vi "Periodic Tasks.vi"(8 "error in":errorcluster) -> ()   [LabVIEW 2016]
doc: "This VI runs in parallel to other tasks. It can contain as many user-defined periodic loops as you need. These can carry out PID or other sorts of timed response."
uses:
  <vilib>/Rock Robotics/WPI/ThirdParty/CanMotor/TalonSRX/WPI_CANTalonSRX_GlobalOps.ctl
  <vilib>/Rock Robotics/WPI/Utilities/WPI_GetSetVariantRefNum.vi
  Robot Global Data.vi
  <vilib>/Rock Robotics/Network Tables/NT Write String Array.vi
  <vilib>/Rock Robotics/Network Tables/NT Write Numeric Array.vi
  2039lib.lvlib
  <vilib>/Rock Robotics/Network Tables/NT Write Number.vi
  <vilib>/Analysis/NI_AALPro.lvlib
  <vilib>/Analysis/2dsp.llb/Integral Method.ctl
  <vilib>/Analysis/8numeric.llb/1D Numeric Integration.vi
panel:
  in  "Auto Names":string[](array[string])
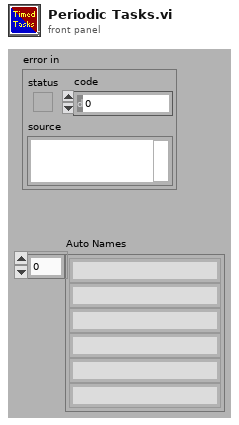
[diagram p1: front panel]
types:
  T1 = typedef "WPI_JoystickDevRef.ctl" = cluster{"Device":T2}
  T2 = typedef "WPI_JoystickDeviceEnum.ctl" = enum16{"USB 0", "USB 1", "USB 2", "USB 3", "USB 4", "USB 5"}
  T3 = typedef "WPI_RobotDriveDevRef.ctl" = cluster{"DevStatus":errorcluster, "Motors[]":T4[], "Square Inputs":bool, "Max Output":dbl}
  T4 = typedef "WPI_MotorControlDeviceRef.ctl" = cluster{"DeviceStatus":errorcluster, "Type":T5, "PWM":cluster{"PWM Channel":T6, "DeadBand":T7}, "CAN":cluster{"Device Number":u8, "SetOutput VI Ref":variant, "GetOutput VI Ref":variant, "Enable VI Ref":variant, "Disable VI Ref":variant, "Data":variant}, "Invert":bool}
  T5 = typedef "WPI_MotorControlType.ctl" = enum16{"PWM", "CAN"}
  T6 = typedef "FPGA_DIOPWMChannel.ctl" = enum8{"PWM 0", "PWM 1", "PWM 2", "PWM 3", "PWM 4", "PWM 5", "PWM 6", "PWM 7", "PWM 8", "PWM 9", "PWM MXP 0", "PWM MXP 1", "PWM MXP 2", "PWM MXP 3", "PWM MXP 4", "PWM MXP 5", "PWM MXP 6", "PWM MXP 7", "PWM MXP 8", "PWM MXP 9", "Invalid"}
  T7 = typedef "WPI_PWMDeadband.ctl" = cluster{"Name":string, "maxPositivePwm":i32, "minPositivePwm":i32, "centerPwm":i32, "maxNegativePwm":i32, "minNegativePwm":i32, "angularRange":u16}
  T8 = cluster{"JoystickDevRef":T1, "RobotDriveDevRef":T3}
  T9 = typedef "NI_AALPro.lvlib/Integral Method.ctl" = i32
  T10 = typedef "WPI_CANTalonSRX_GlobalOps.ctl" = enum16{"Read For Send", "Write After Receive General", "Write After Receive Feedback", "Write After Receive Encoder", "Write After Receive Ain", "Write Error", "Get All", "Set Output", "Set Mode", "Set Master ID", "Set Brake Mode", "Set Reverse Feedback Sensor", "Set Reverse Closed Loop Output", "Set Override Limits", "Set Forward Limit Enabled", "Set Reverse Limit Enabled", "Set Feedback Select", "Set Profile Select", "Set Throttle Ramp Rate", "Disable", "Set Enc Codes Per Rev", "Set Num Pot Turns", "Set Control Frame Rate", "Enable Legacy Control", "Write After Receive Pulse Width", "Set Enable Frame Rate", "Write After Receive Motion Profile", "Set Motion Profile Flow Control", "Set Motion Profile Control Frame Rate", "Set Current Limit Enable", "Set Usage Frame"}
  T11 = typedef "WPI_CANTalonSRX_GlobalStatus.ctl" = cluster{"Applied Throttle":dbl, "Module Enabled":bool, "CAN Error":errorcluster, "Closed Loop Error":dbl, "Forward Limit Switch Closed":bool, "Reverse Limit Switch Closed":bool, "Sensor Position":dbl, "Sensor Velocity":dbl, "Current":dbl, "Sticky Fault - Over Temp":bool, "Sticky Fault - Under Voltage":bool, "Sticky Fault - Forward Limit":bool, "Sticky Fault - Reverse Limit":bool, "Sticky Fault - Forward Soft Limit":bool, "Sticky Fault - Reverse Soft Limit":bool, "Brake is Enabled":bool, "Encoder Position":dbl, "Encoder Velocity":dbl, "Encoder Index Count":dbl, "Encoder A Pin State":bool, "Encoder B Pin State":bool, "Encoder Index Pin State":bool, "Analog In":dbl, "Analog In Velocity":dbl, "Temperature (C)":dbl, "Battery Voltage":dbl, "Control 5 Is Supported":bool, "Current Profile Slot Select":dbl, "Pos Div 8":bool, "Vel Div 4":bool, "Pulse Width Position":i32, "Pulse Width Velocity":i32, "Pulse Width Rise To Rise (us)":i32, "Pulse Width Rise To Fall (us)":i32, "Mot Prof Active Is Under Run":bool, "Mot Prof Active Has Under Run":bool, "Mot Prof Active Is Last":bool, "Mot Prof Active Velocity Only":bool, "Mot Prof Active Is Valid":bool, "Mot Prof Buffer Is Full":bool, "Mot Prof Active Profile Slot Select":i32, "Mot Prof NextID":i32, "Mot Prof Count":i32, "Mot Prof Active Velocity":dbl, "Mot Prof Active Position":dbl, "Mot Prof Output Enable":i32, "UsageFrame":u32}
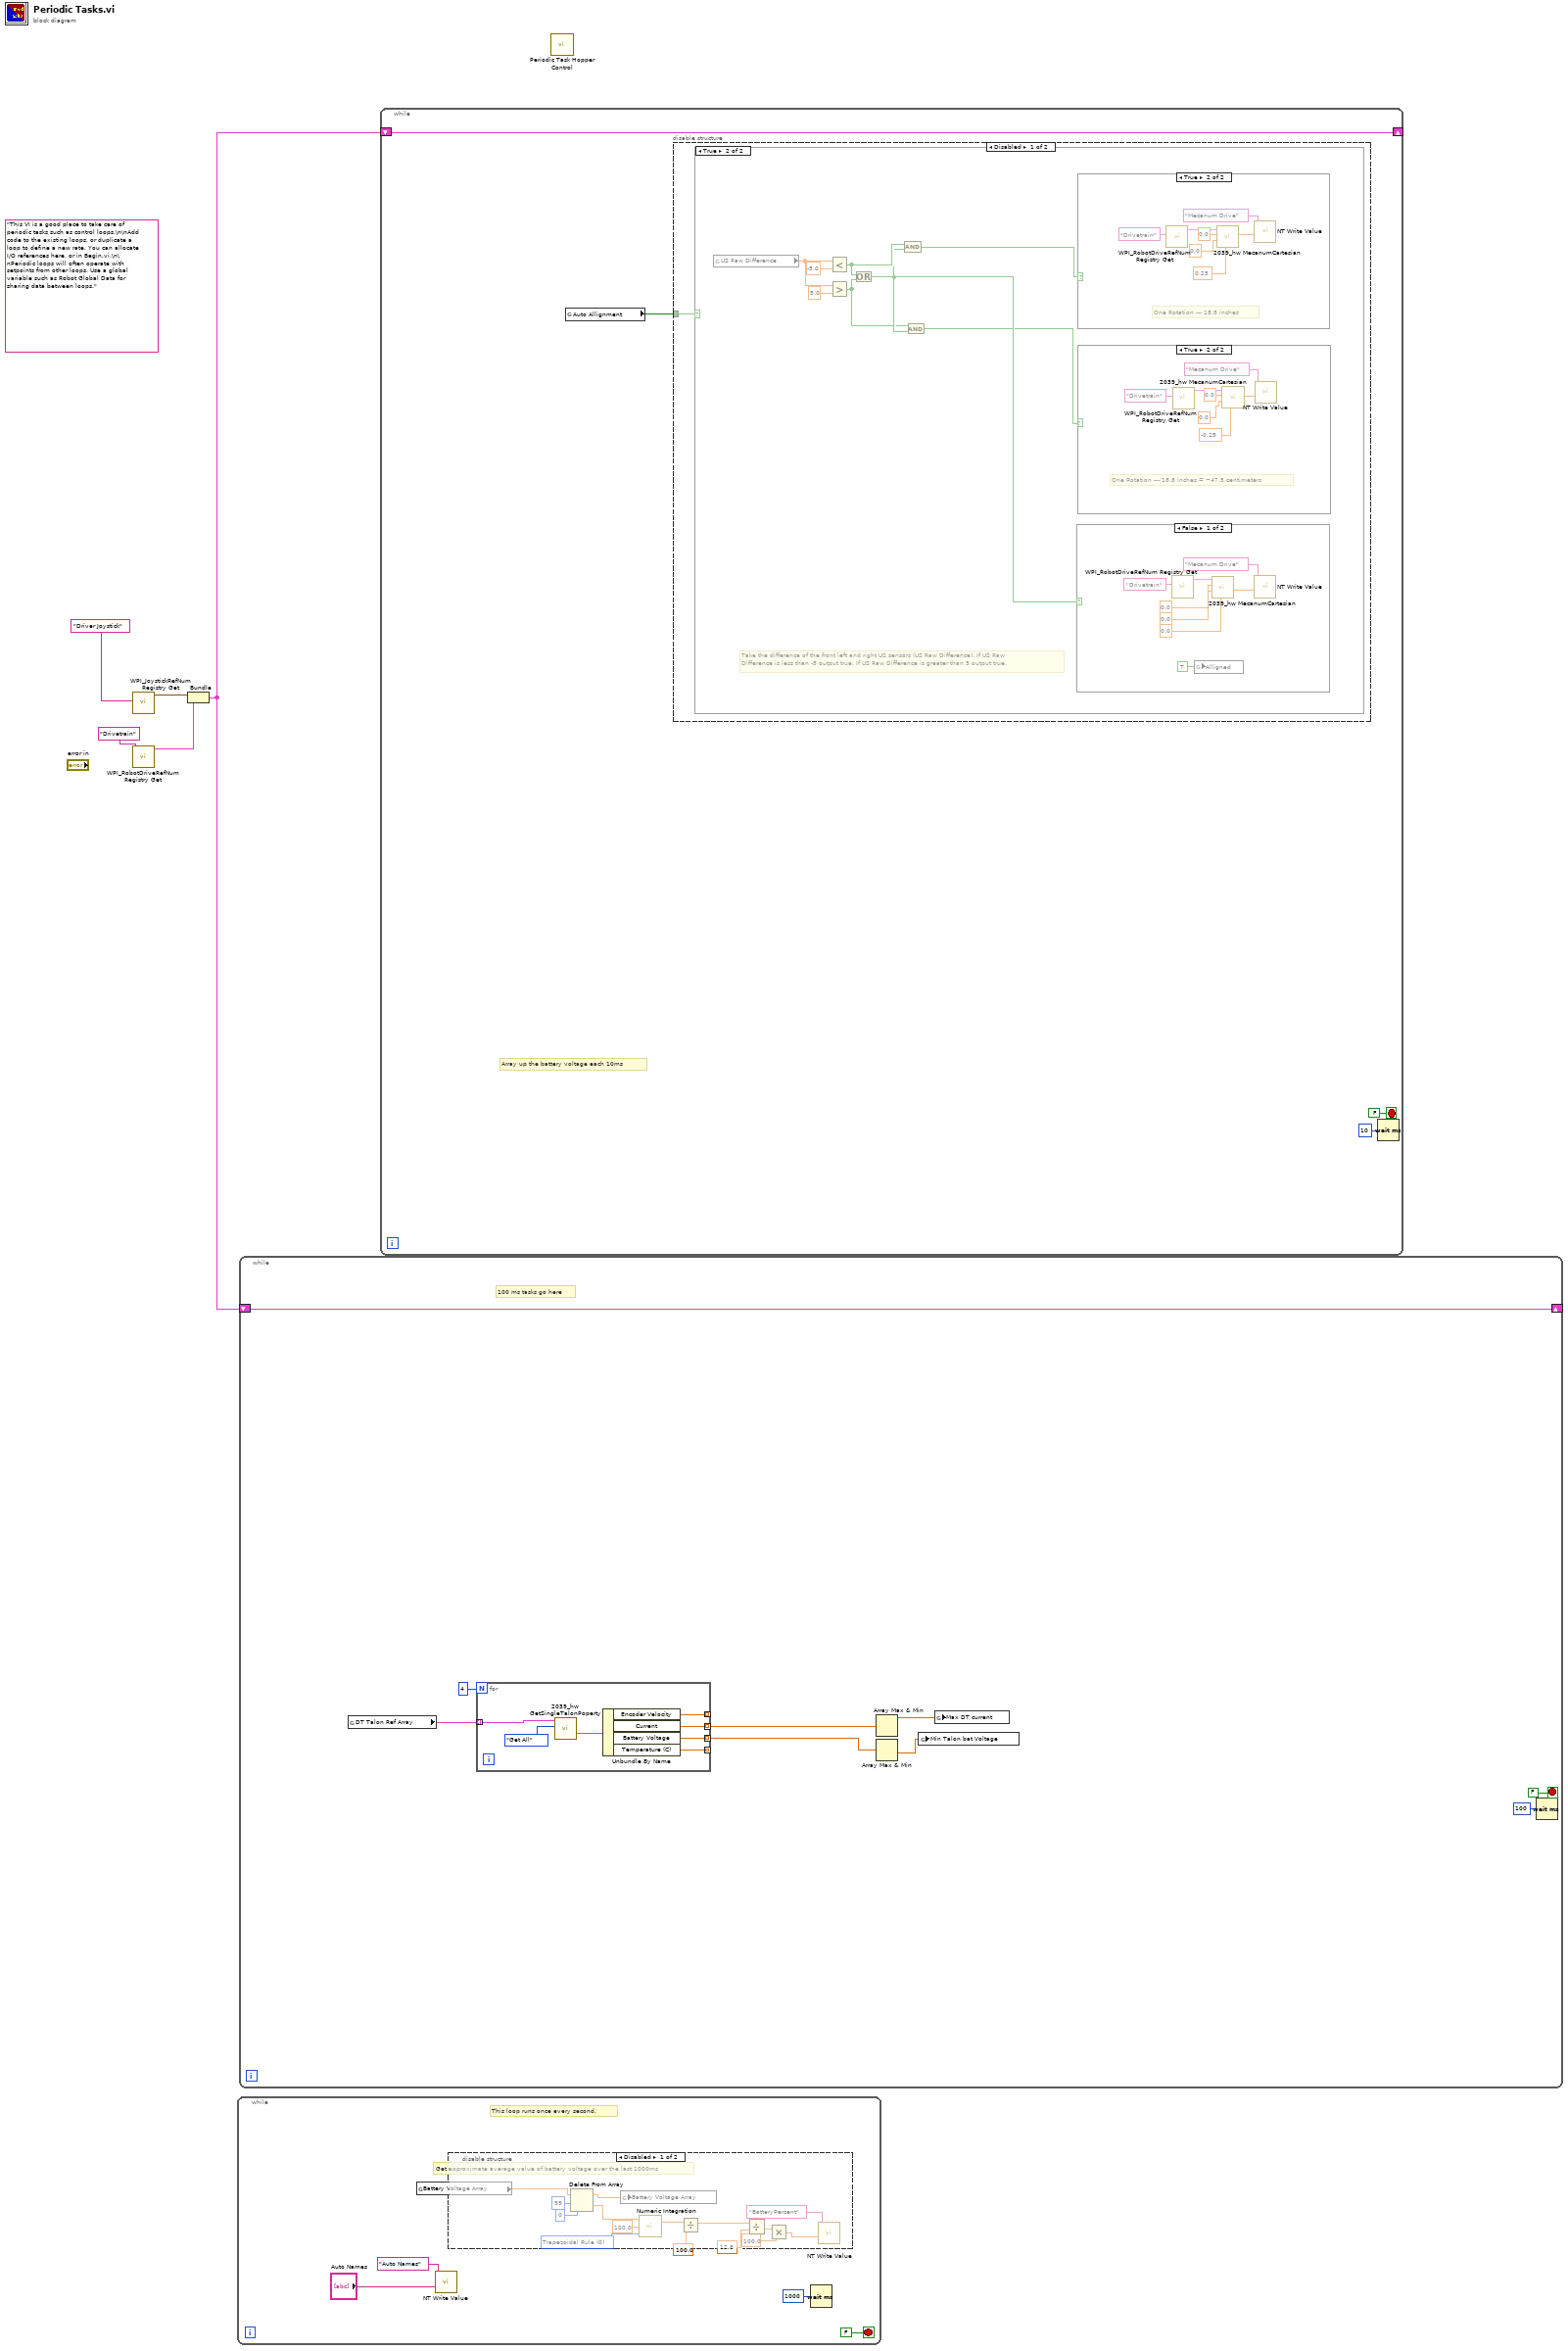
[diagram p0: block diagram]
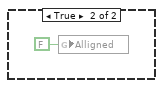
[diagram p4: hidden frame]
diagram:
  (unwired) "This VI is a good place to take care of periodic tasks such as control loops.\n\nAdd code to the existing loops, or duplicate a loop to define a new rate. You can allocate I/O references here, or in Begin.vi.\n\nPeriodic loops will often operate with setpoints from other loops. Use a global variable such as Robot Global Data for sharing data between loops."
  n1 = call <vilib>:"WPI_JoystickRefNum Registry Get.vi"("refnum name"="Driver Joystick") -> ("JoystickDevRef"=w3:T1)  [unwired: 1 in, 9 out]
  n2 = call <vilib>:"WPI_RobotDriveRefNum Registry Get.vi"("refnum name"="Drivetrain") -> ("RobotDriveDevRef"=w2:T3)  [unwired: 1 in, 9 out]
  n3 = Bundle("JoystickDevRef"=w3, "RobotDriveDevRef"=w2) -> (w1:T8)  [unwired: 1 out]
  n4 = while {
    stop <- FALSE stop-if-true
    # "This loop runs once every second."
    n5 = call-poly <vilib>:"NT Write Value.vi"("String Array"="Auto Names", "Name"="Auto Names") -> ()  [unwired: 9 in, 1 out]
    n6 = disable-structure shown="Disabled" {
      frame Disabled {
        w21 = T9 0 items=["Trapezoidal Rule", "Simpson's Rule", "Simpson's 3/8 Rule", "Bode Rule"] ("integration method")
        # "Get approximate average value of battery voltage over the last 1000ms"
        n7 = global read "Robot Global Data.vi" "Battery Voltage Array"() -> (w16:dbl[])
        n8 = Delete From Array(array=w16, length=99, index=0) -> (deleted portion=w20:dbl[], array with subset deleted=w19:dbl[])
        n9 = global write "Robot Global Data.vi" "Battery Voltage Array"(w19) -> ()
        n10 = call-poly <vilib>:"Numeric Integration.vi"("integration method"=w21, "dt"=100.0, "Input Array"=w20) -> ("result"=w23:dbl)  [unwired: 1 out]
        n11 = Divide(x=w23, y=100.0) -> (x/y=w15:dbl)
        n12 = Divide(x=w15, y=12.8) -> (x/y=w13:dbl)
        n13 = Multiply(x=w13, y=100.0) -> (x*y=w11:dbl)
        n14 = call-poly <vilib>:"NT Write Value.vi"("Numeric"=w11, "Name"="BatteryPercent") -> ()  [unwired: 9 in, 1 out]
      }
      frame Enabled {
      }
    }
    n15 = Wait (ms)(milliseconds to wait=u32 1000) -> ()  [unwired: 1 out]
  }
  n16 = while {
    shift-right: [w31] -> _
    shift-left: w1 -> [w31]
    stop <- FALSE stop-if-true
    # "100 ms tasks go here"
    n17 = global read "Robot Global Data.vi" "DT Talon Ref Array"() -> (w29:T4[])
    n18 = for {
      N: 4 -> [_]
      tunnel: w29 -> [w40] mode=indexing
      tunnel: [w37] -> w28 mode=indexing
      tunnel: [w36] -> _ mode=indexing
      tunnel: [w35] -> w26 mode=indexing
      tunnel: [w34] -> _ mode=indexing
      n19 = call "2039_hw GetSingleTalonPoperty.vi"("Operation"=WPI_CANTalonSRX_GlobalOps."Get All", "CAN Talon SRX Ref"=w40) -> ("Talon SRX Status"=w38:T11)  [unwired: 7 in, 2 out]
      n20 = Unbundle By Name(w38) -> ("Encoder Velocity"=w36:dbl, "Current"=w37:dbl, "Battery Voltage"=w35:dbl, "Temperature (C)"=w34:dbl)
    }
    n21 = Array Max & Min(array=w28) -> (max value=w27:dbl)  [unwired: 3 out]
    n22 = Array Max & Min(array=w26) -> (min value=w25:dbl)  [unwired: 3 out]
    n23 = global write "Robot Global Data.vi" "Min Talon bat Voltage"(w25) -> ()
    n24 = global write "Robot Global Data.vi" "Max DT current"(w27) -> ()
    n25 = Wait (ms)(milliseconds to wait=u32 100) -> ()  [unwired: 1 out]
  }
  n26 = while {
    shift-right: [w42] -> _
    shift-left: w1 -> [w42]
    stop <- FALSE stop-if-true
    # "Array up the battery voltage each 10ms"
    n27 = global read "Robot Global Data.vi" "Auto Allignment"() -> (w41:bool)
    n28 = disable-structure shown="Disabled" {
      disable-tunnel: w41 -> [w45 _]
      frame Disabled {
        n29 = case shown="True" w45 {
          frame False {
          }
          frame True {
            # "Take the difference of the front left and right US sensors (US Raw Difference). If US Raw \nDifference is less than -5 output true. If US Raw Difference is greater than 5 output true."
            n30 = global read "Robot Global Data.vi" "US Raw Difference"() -> (w51:dbl)
            n31 = Less?(x=w51, y=-5.0) -> (x < y?=w50:bool)
            n32 = Greater?(x=w51, y=5.0) -> (0:w47:bool)
            n33 = Or(x=w50, y=w47) -> (x .or. y?=w48:bool)
            n34 = And(x=w50, y=w48) -> (x .and. y?=w49:bool)
            n35 = And(x=w47, y=w48) -> (x .and. y?=w46:bool)
            n36 = case shown="False" w48 {
              frame False {
                n37 = call <vilib>:"WPI_RobotDriveRefNum Registry Get.vi"("refnum name"="Drivetrain") -> ("RobotDriveDevRef"=w59:T3)  [unwired: 9 in, 1 out]
                n38 = global write "Robot Global Data.vi" "Alligned"(TRUE ("Alligned")) -> ()
                n39 = call "2039_hw MecanumCartesian.vi"("Rotation"=0.0, "Y"=0.0, "X"=0.0, "RobotDriveDevRef"=w59) -> ("Motor Values"=w60:dbl[])  [unwired: 5 in, 2 out]
                n40 = call-poly <vilib>:"NT Write Value.vi"("Numeric Array"=w60, "Name"="Mecanum Drive") -> ()  [unwired: 9 in, 1 out]
              }
              frame True {
                n41 = global write "Robot Global Data.vi" "Alligned"(FALSE ("Alligned")) -> ()
              }
            }
            n42 = case shown="True" w46 {
              frame False {
              }
              frame True {
                # "One Rotation --- 18.8 inches = ~47.5 centimeters"
                n43 = call <vilib>:"WPI_RobotDriveRefNum Registry Get.vi"("refnum name"="Drivetrain") -> ("RobotDriveDevRef"=w67:T3)  [unwired: 9 in, 1 out]
                n44 = call "2039_hw MecanumCartesian.vi"("Rotation"=-0.25 ("X"), "Y"=0.0 ("X"), "X"=0.0, "RobotDriveDevRef"=w67) -> ("Motor Values"=w68:dbl[])  [unwired: 5 in, 2 out]
                n45 = call-poly <vilib>:"NT Write Value.vi"("Numeric Array"=w68, "Name"="Mecanum Drive") -> ()  [unwired: 9 in, 1 out]
              }
            }
            n46 = case shown="True" w49 {
              frame False {
              }
              frame True {
                # "One Rotation --- 18.8 inches"
                n47 = call <vilib>:"WPI_RobotDriveRefNum Registry Get.vi"("refnum name"="Drivetrain") -> ("RobotDriveDevRef"=w74:T3)  [unwired: 9 in, 1 out]
                n48 = call "2039_hw MecanumCartesian.vi"("Rotation"=0.25 ("X"), "Y"=0.0 ("X"), "X"=0.0, "RobotDriveDevRef"=w74) -> ("Motor Values"=w75:dbl[])  [unwired: 5 in, 2 out]
                n49 = call-poly <vilib>:"NT Write Value.vi"("Numeric Array"=w75, "Name"="Mecanum Drive") -> ()  [unwired: 9 in, 1 out]
              }
            }
          }
        }
      }
      frame Enabled {
      }
    }
    n50 = Wait (ms)(milliseconds to wait=u32 10) -> ()  [unwired: 1 out]
  }
  n51 = call "Periodic Task Hopper Control.vi"() -> ()  [unwired: 12 in]
